vi "Connect_test.vi"() -> ()   [LabVIEW 2020]
uses:
  C:/Program Files/Metrohm Autolab/Autolab SDK 2.1/EcoChemie.Autolab.Sdk.dll
  Program Files/Metrohm Autolab/Autolab SDK 2.1/EcoChemie.Autolab.Sdk.dll
  Autolab dependencies/TypeDef.ctl
panel:
  in  "Initalising Current range":i32(ring)=-3 items=["CR07_1A"=0, "CR06_10A"=1, "CR01_100A"=2, "CR00_1000A"=3, "CR05_20A"=20, "CR04_40A"=40, "CR03_50A"=60, "CR02_80A"=80, "CR19_1pA"=-12, "CR18_10pA"=-11, "CR17_100pA"=-10, "CR16_1nA"=-9, "CR15_10nA"=-8, "CR14_100nA"=-7, "CR13_1uA"=-6, "CR12_10uA"=-5, "CR11_100uA"=-4, "CR10_1mA"=-3, "CR09_10mA"=-2, "CR08_100mA"=-1]
  in  "Connect only?":bool=TRUE
  out "error after Ei":errorcluster
  out "after conect":errorcluster
  in  "Embedded Exe File":path=path "C:/Users/Benj/Desktop/Autolab software stuff/Minimal working example/Adk.x"
  out "Ei":refnum<k24>
  out "Sampler 2":refnum<k24>
  out "AutolabConnection":refnum<k24>
  out "Dio":refnum<k24>
  out "Dac":refnum<k24>
  out "Adc":refnum<k24>
  out "instrument":refnum<k24>
  in  "Hardware Setup File":path=path "C:/Users/Benj/Desktop/Autolab software stuff/Minimal working example/HardwareSetup.AUT55157.xml"
  in  "read continually?":bool
  out "Setpoint":dbl
  out "Mode":i32(ring) items=["Potentiostatic", "Galvanostatic"]
  out "CurrentRange":i32(ring) items=["CR07_1A"=0, "CR06_10A"=1, "CR01_100A"=2, "CR00_1000A"=3, "CR05_20A"=20, "CR04_40A"=40, "CR03_50A"=60, "CR02_80A"=80, "CR19_1pA"=-12, "CR18_10pA"=-11, "CR17_100pA"=-10, "CR16_1nA"=-9, "CR15_10nA"=-8, "CR14_100nA"=-7, "CR13_1uA"=-6, "CR12_10uA"=-5, "CR11_100uA"=-4, "CR10_1mA"=-3, "CR09_10mA"=-2, "CR08_100mA"=-1]
  out "Bandwidth":i32(ring) items=["UltraHigh_Speed", "High_Speed", "High_Stability"]
  out "EI status supported for":string[](array[string])
  in  "Bandwidth 2":i32(ring)=2 items=["UltraHigh_Speed", "High_Speed", "High_Stability"]
  in  "CellOnOff":i32(ring) items=["Off", "On"]
  in  "Mode 2":i32(ring) items=["Potentiostatic", "Galvanostatic"]
  in  "Setpoint 2":dbl
  out "Oscillation":bool
  out "Current":dbl
  out "PotentialOverload":bool
  out "CurrentOverload":bool
  out "ManualCellSwitch":bool
  out "TemperatureOverload":bool
  out "Cell":bool
  out "Potential":dbl
  # "Note: Adk.x must be in\nC:\\Program Files\\Metrohm Autolab\\Autolab SDK 2.1\\Hardware Setup Files\\Adk.x"
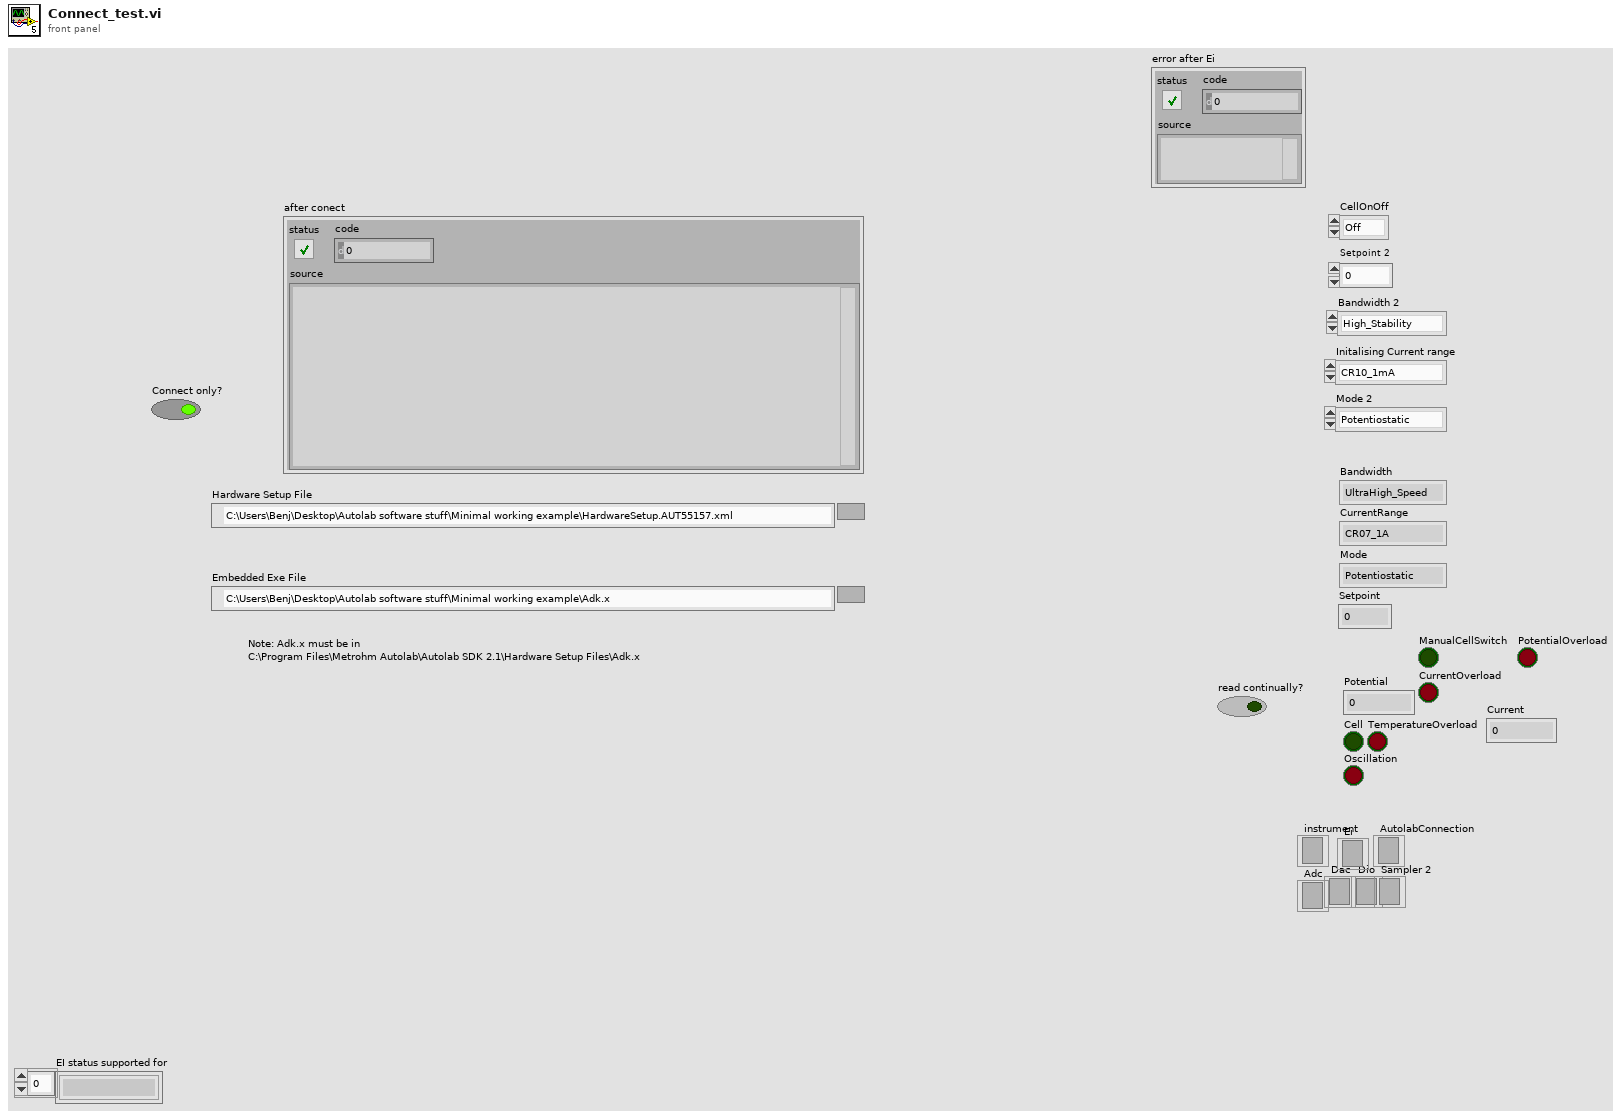
[diagram p1: front panel]
types:
  T1 = typedef "TypeDef.ctl" = enum16{"Connect", "Read", "End"}
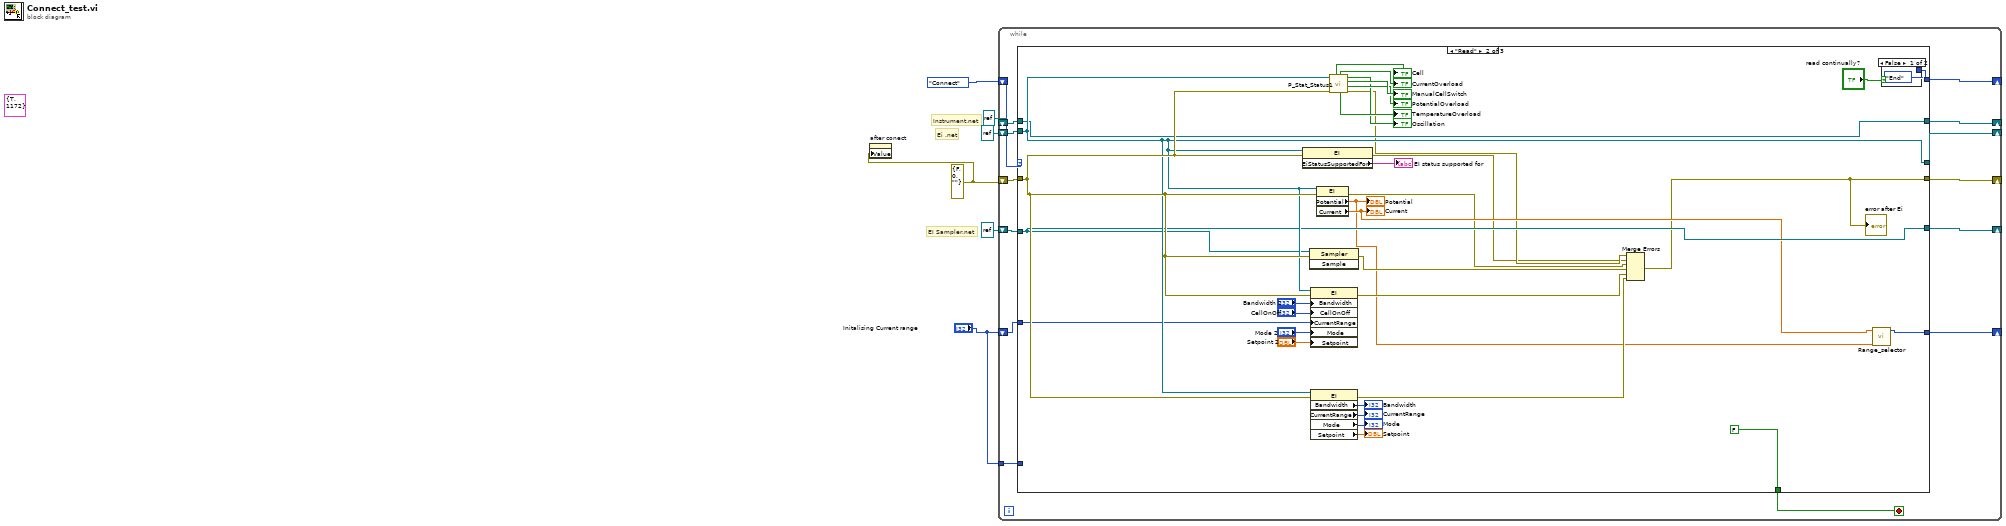
[diagram p0: block diagram]
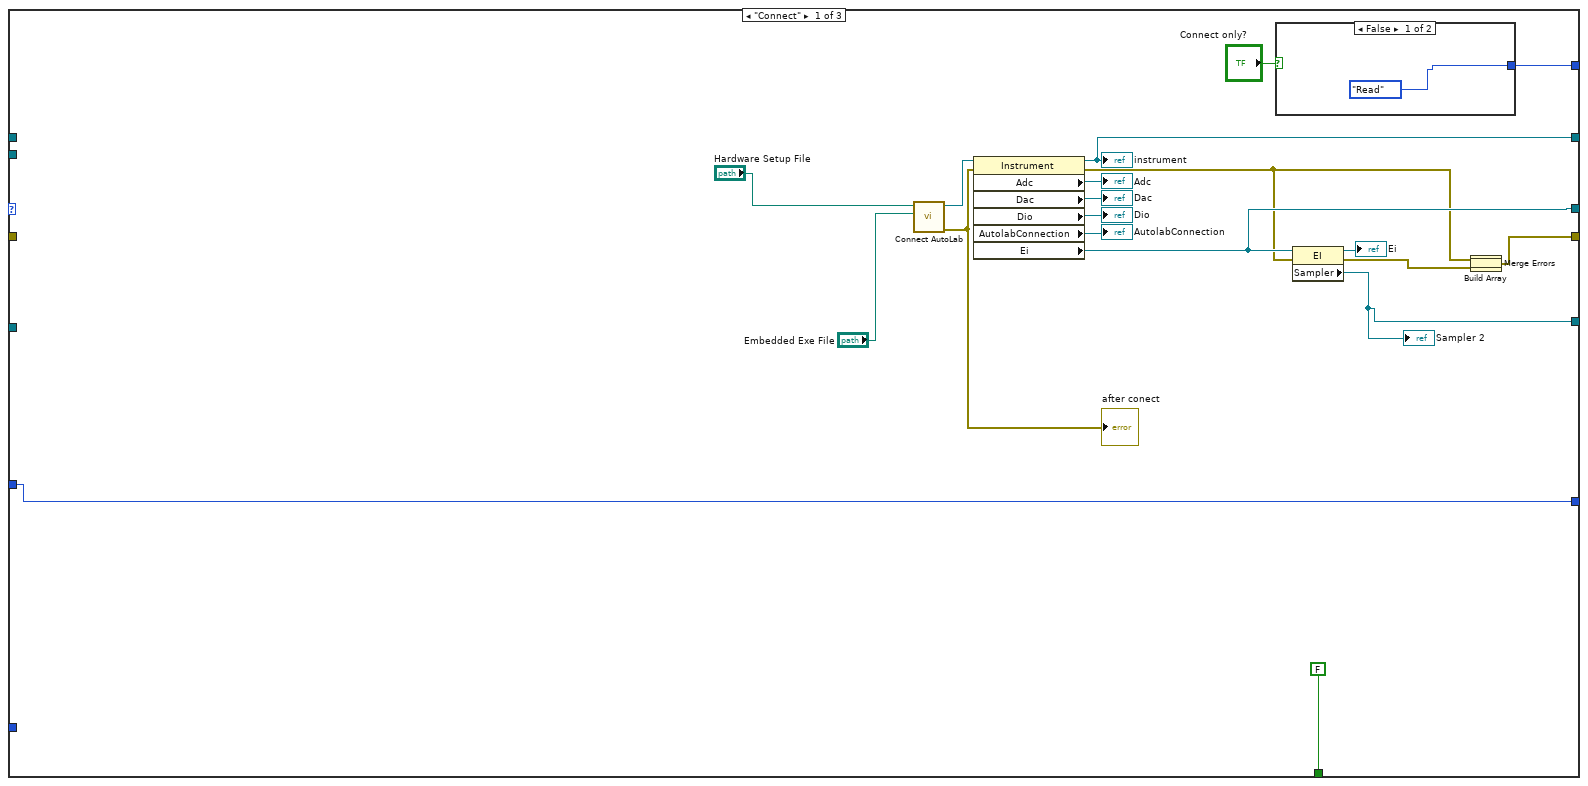
[diagram p2: hidden frame]
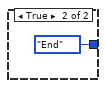
[diagram p3: hidden frame]
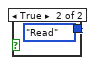
[diagram p4: hidden frame]
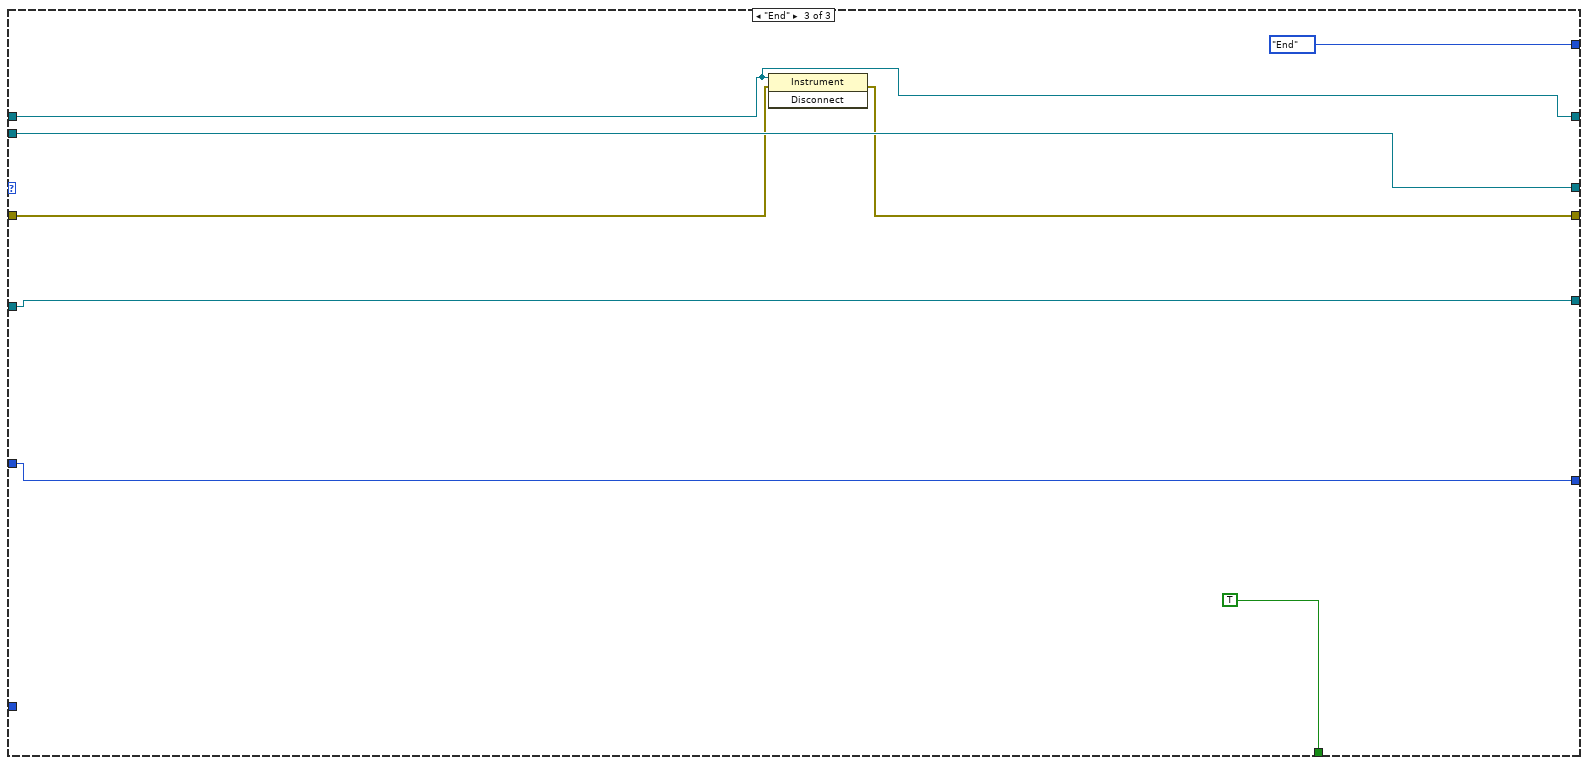
[diagram p5: hidden frame]
diagram:
  (unwired) cluster{"status":bool, "code":i32} {"status"=TRUE, "code"=1172} ("Error after connect")
  w3 = errorcluster {"status"=FALSE, "code"=0, "source"=""} ("error in (no error)")
  # "Instrument.net"
  # "EI Sampler.net"
  # "Ei .net"
  n1 = property on="after conect" class="Clust (strict)"("Value"=w3) -> ()  [unwired: 2 in, 2 out]
  n2 = while {
    shift-right: [w14] -> _
    shift-left: refnum<k24> refnum ("Ei") -> [w15]
    shift-right: [w17] -> _
    shift-left: w3 -> [w18]
    shift-right: [w19] -> _
    shift-left: TypeDef."Connect" -> [w20]
    shift-right: [w13] -> _
    shift-left: refnum<k24> refnum ("Sampler") -> [w12]
    shift-right: [w11] -> _
    shift-left: refnum<k24> refnum ("new reference") -> [w10]
    shift-right: [w9] -> _
    shift-left: "Initalising Current range" -> [w8]
    tunnel: "Initalising Current range" -> [w7]
    stop <- w16 stop-if-true
    n3 = case shown="\"Read\"" w20 {
      tunnel: [w27 w67 w84] -> w14
      tunnel: [w40 w75 TypeDef."End"] -> w19
      tunnel: w18 -> [_ w69 w80]
      tunnel: [w28 w44 w79] -> w17
      tunnel: [FALSE FALSE TRUE] -> w16
      tunnel: w15 -> [_ w67 w84]
      tunnel: [w24 w65 w82] -> w13
      tunnel: w12 -> [_ w65 w82]
      tunnel: [w23 w60 w81] -> w11
      tunnel: w10 -> [_ w60 w81]
      tunnel: w8 -> [w21 w59 w78]
      tunnel: [w21 w57 w78] -> w9
      tunnel: w7 -> [_ _ _]
      frame "Connect" {
        n4 = call "Connect AutoLab.vi"("Embedded Exe File"="Embedded Exe File", "Hardware Setup File"="Hardware Setup File") -> ("error out"=w25:errorcluster, ".NET Refnum out"=w37:refnum<k24>)  [unwired: 8 in]
        "after conect" <- w25
        n5 = property class="Instrument"(reference=w37, error in=w25) -> (reference out=w23:refnum<k24>, error out=w26:errorcluster, "Adc"=→"Adc":refnum<k24>, "Dac"=→"Dac":refnum<k24>, "Dio"=→"Dio":refnum<k24>, "AutolabConnection"=→"AutolabConnection":refnum<k24>, "Ei"=w27:refnum<k24>)
        "instrument" <- w23
        n6 = case shown="False" "Connect only?" {
          tunnel: [TypeDef."Read" TypeDef."End"] -> w40
          frame False {
          }
          frame True {
          }
        }
        n7 = property class="EI"(reference=w27, error in=w26) -> (reference out=→"Ei":refnum<k24>, error out=w36:errorcluster, "Sampler"=w24:refnum<k24>)
        "Sampler 2" <- w24
        n8 = Build Array(w26, w36) -> (w29:errorcluster[])
        n9 = Merge Errors(w29) -> (w28:errorcluster)
      }
      frame "Read" {
        n10 = property class="EI"(reference=w67, error in=w69) -> (error out=w49:errorcluster, "EiStatusSupportedFor"=→"EI status supported for":string[])  [unwired: 1 out]
        n11 = invoke class="Sampler" method="Sample"(reference=w65, error in=w69) -> (error out=w47:errorcluster)  [unwired: 1 in, 2 out]
        n12 = property class="EI"(reference=w67, error in=w69, "Bandwidth"="Bandwidth 2", "CellOnOff"="CellOnOff", "CurrentRange"=w59, "Mode"="Mode 2", "Setpoint"="Setpoint 2") -> (error out=w46:errorcluster)  [unwired: 1 out]
        n13 = property class="EI"(reference=w67, error in=w69) -> (error out=w45:errorcluster, "Bandwidth"=→"Bandwidth":i32, "CurrentRange"=→"CurrentRange":i32, "Mode"=→"Mode":i32, "Setpoint"=→"Setpoint":dbl)  [unwired: 1 out]
        n14 = property class="EI"(reference=w67, error in=w69) -> (error out=w48:errorcluster, "Potential"=w43:dbl, "Current"=w58:dbl)  [unwired: 1 out]
        "Potential" <- w43
        "Current" <- w58
        n15 = call "P_Stat_Status1.vi"("error in (no error)"=w69, ".NET Refnum in"=w67) -> ("error out"=w50:errorcluster, "PotentialOverload"=→"PotentialOverload":bool, "ManualCellSwitch"=→"ManualCellSwitch":bool, "Oscillation"=→"Oscillation":bool, "TemperatureOverload"=→"TemperatureOverload":bool, "CurrentOverload"=→"CurrentOverload":bool, "Cell"=→"Cell":bool)  [unwired: 3 in]
        n16 = Merge Errors(w50, w49, w48, w47, w46, w45) -> (w44:errorcluster)
        "error after Ei" <- w44
        n17 = call "Range_selector.vi"("potential"=w43, "current"=w58) -> ("range integer"=w57:i32)  [unwired: 9 in]
        n18 = case shown="False" "read continually?" {
          tunnel: [TypeDef."End" TypeDef."Read"] -> w75
          frame False {
          }
          frame True {
          }
        }
      }
      frame "End" {
        n19 = invoke class="Instrument" method="Disconnect"(reference=w81, error in=w80) -> (error out=w79:errorcluster)  [unwired: 1 in, 2 out]
      }
    }
  }
